vi "Revision Query.vi"(8 "error in (no error)":errorcluster, 11 "VISA resource name":refnum<visa-resource-name>) -> (0 "error out":errorcluster, 1 "Instrument Firmware Revision":string, 2 "Instrument Driver Revision":string, 3 "VISA resource name out":refnum<visa-resource-name>)   [LabVIEW 2016, in "MGC647C.lvlib"]
doc: "Queries the current instrument firmware revision and instrument driver revision.\n\nRefer to the Readme file for detailed driver information including modification history."
uses:
  MGC647C.lvlib
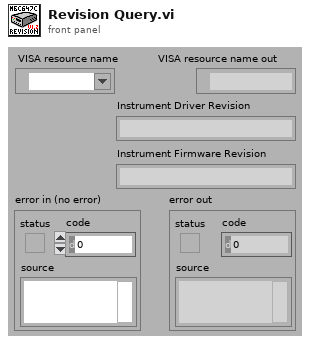
[diagram p1: front panel]
types:
  T1 = cluster{"Major":u16, "Minor":u16, "Fix":u16, "Build":u16}
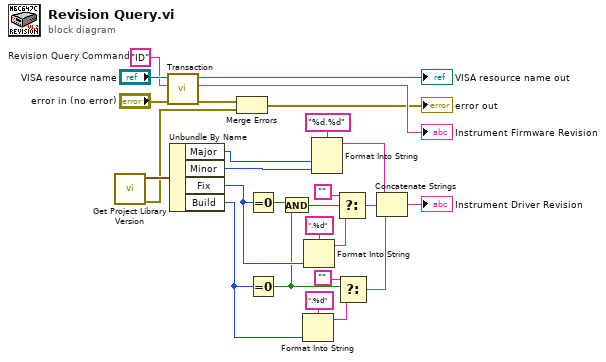
[diagram p0: block diagram]
diagram:
  w25 = "ID"  # Revision Query Command
  n1 = call <vilib>:"Get Project Library Version.vi"() -> ("error out"=w3:errorcluster, "Project Library Version"=w5:T1)  [unwired: 10 in]
  n2 = call "Transaction.vi"("Error In"="error in (no error)", "Command"=w25, "VISA resource name"="VISA resource name") -> ("Error Out"=w2:errorcluster, "Response"=→"Instrument Firmware Revision":string, "dup VISA resource name"=→"VISA resource name out":refnum<visa-resource-name>)  [unwired: 6 in]
  n3 = Unbundle By Name(w5) -> ("Major"=w12:u16, "Minor"=w11:u16, "Fix"=w9:u16, "Build"=w10:u16)
  n4 = Merge Errors(w2, w3) -> (→"error out":errorcluster)
  n5 = Equal To 0?(x=w9) -> (x = 0?=w8:bool)
  n6 = Equal To 0?(x=w10) -> (x = 0?=w7:bool)
  n7 = And(x=w8, y=w7) -> (x .and. y?=w6:bool)
  n8 = Format Into String(format string=".%d", w10) -> (resulting string=w16:string)  [unwired: 2 in, 1 out]
  n9 = Format Into String(format string=".%d", w9) -> (resulting string=w20:string)  [unwired: 2 in, 1 out]
  n10 = Format Into String(format string="%d.%d", w12, w11) -> (resulting string=w18:string)  [unwired: 2 in, 1 out]
  n11 = Select(t="", s=w6, f=w20) -> (s? t:f=w17:string)
  n12 = Select(t="", s=w7, f=w16) -> (s? t:f=w13:string)
  n13 = Concatenate Strings(w18, w17, w13) -> (→"Instrument Driver Revision":string)
